vi "Compute Convolution 32f.vi"(8 "Error In":errorcluster, 10 "Input Memory":T4 {"Dimension"."Width" min=1; "Dimension"."Height" min=1; "Dimension"."Depth" min=1}, 11 "Convolution Object":T1 {"Convolved Memory Object"."Dimension"."Width" min=1; "Convolved Memory Object"."Dimension"."Height" min=1; "Convolved Memory Object"."Dimension"."Depth" min=1; "Kernel Memory Object"."Dimension"."Width" min=1; "Kernel Memory Object"."Dimension"."Height" min=1; "Kernel Memory Object"."Dimension"."Depth" min=1}) -> (0 "Error Out":errorcluster, 2 "Convolved Memory":T4 {"Dimension"."Width" min=1; "Dimension"."Height" min=1; "Dimension"."Depth" min=1}, 3 "Convolution Object Out":T1 {"Convolved Memory Object"."Dimension"."Width" min=1; "Convolved Memory Object"."Dimension"."Height" min=1; "Convolved Memory Object"."Dimension"."Depth" min=1; "Kernel Memory Object"."Dimension"."Width" min=1; "Kernel Memory Object"."Dimension"."Height" min=1; "Kernel Memory Object"."Dimension"."Depth" min=1}, 4 "Time in ms":dbl)   [LabVIEW 2012, in "OpenCLV x64.lvlib"]
doc: "Convolves the input memory object with the kernel that has been previously set. The output is seperate from the input."
uses:
  OpenCLV x64.lvlib
  Controls/Convolution Object.ctl
  Controls/Device ID.ctl
  Controls/Program Handle.ctl
  Controls/Memory Object.ctl
  Controls/Memory ID.ctl
  User Controls/Array Dimensions.ctl
  Controls/Memory Type.ctl
  Error Checking/Add Error Functional Global.vi
  Set Kernel Arguments/Set Kernel Arguments Memory Object.vi
  Set Kernel Arguments/Set Kernel Arguments int.vi
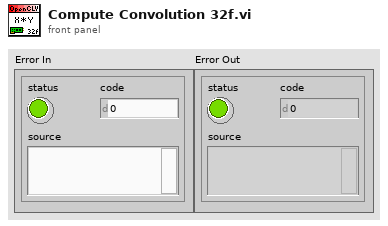
[diagram p1: front panel]
types:
  T1 = typedef "OpenCLV x64.lvlib/Convolution Object.ctl" = cluster{"Device In":T2, "Program Handle":T3, "Kernel Memory Object":T4, "Convolved Memory Object":T4}
  T2 = typedef "OpenCLV x64.lvlib/Device ID.ctl" = u64
  T3 = typedef "OpenCLV x64.lvlib/Program Handle.ctl" = u64
  T4 = typedef "OpenCLV x64.lvlib/Memory Object.ctl" = cluster{"Device ID":T2, "Memeroy ID":T5, "Dimension":T6, "Memory Type":T7}
  T5 = typedef "OpenCLV x64.lvlib/Memory ID.ctl" = u64
  T6 = typedef "Array Dimensions.ctl" = cluster{"Depth":u64, "Height":u64, "Width":u64}
  T7 = typedef "OpenCLV x64.lvlib/Memory Type.ctl" = enum16{"32f", "u8", "i8", "u16", "i16", "u32", "i32", "64f"}
  T8 = typedef "OpenCLV x64.lvlib/Kernel Handle.ctl" = u64
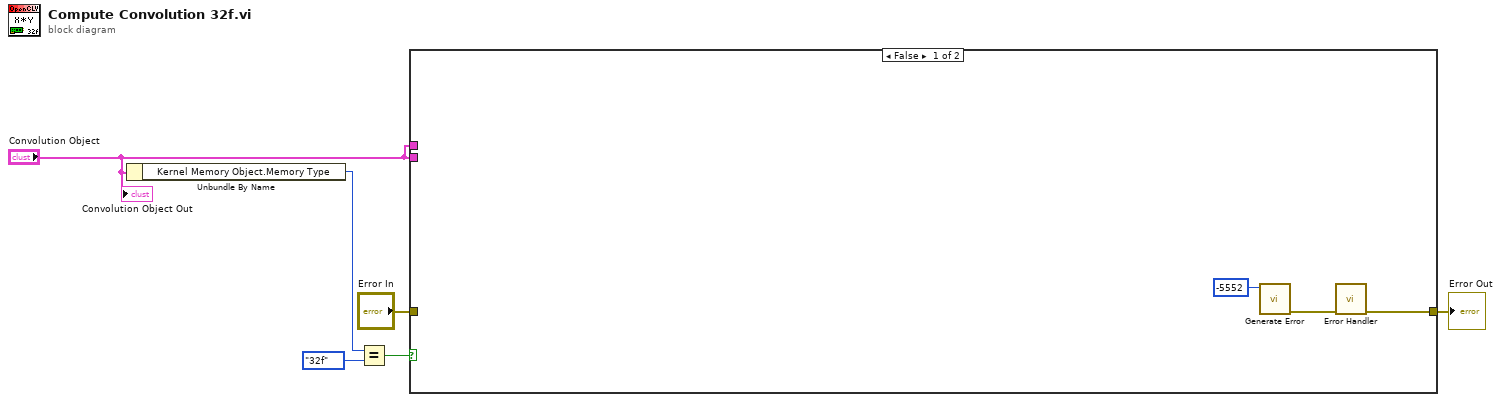
[diagram p0: block diagram]
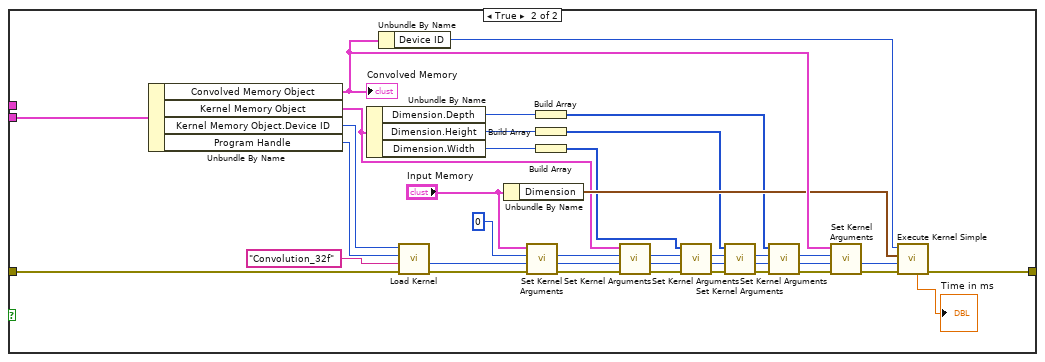
[diagram p2: hidden frame]
diagram:
  n1 = Unbundle By Name("Convolution Object") -> ("Kernel Memory Object.Memory Type"=w6:T7)
  n2 = Equal?(x=w6, y=Memory_Type."32f") -> (x = y?=w5:bool)
  n3 = case shown="False" w5 {
    tunnel: [w7 w46] -> w2
    tunnel: "Convolution Object" -> [_ w36]
    tunnel: "Error In" -> [_ w47]
    tunnel: "Convolution Object" -> [_ _]
    frame False {
      n4 = call "Generate Error.vi"("Error"=-5552) -> ("error out"=w8:errorcluster)  [unwired: 10 in]
      n5 = call-poly "Error Handler.vi"("Error In"=w8) -> ("Error Out"=w7:errorcluster)  [unwired: 10 in]
    }
    frame True {
      n6 = Unbundle By Name(w36) -> ("Convolved Memory Object"=w31:T4, "Kernel Memory Object"=w28:T4, "Kernel Memory Object.Device ID"=w45:T2, "Program Handle"=w35:T3)
      "Convolved Memory" <- w31
      n7 = Unbundle By Name(w28) -> ("Dimension.Depth"=w14:u64, "Dimension.Height"=w19:u64, "Dimension.Width"=w23:u64)
      n8 = Unbundle By Name(w31) -> ("Device ID"=w30:T2)
      n9 = call "Load Kernel.vi"("Error In"=w47, "Kernel Name"="Convolution_32f", "Program Handle"=w35, "Device In"=w45) -> ("Error Out"=w43:errorcluster, "Kernel Handle"=w42:T8)  [unwired: 4 in, 2 out]
      n10 = Unbundle By Name("Input Memory") -> ("Dimension"=w29:T6)
      n11 = call-poly "Set Kernel Arguments.vi"("Error In"=w43, "Kernel Handle"=w42, "Argument Number"=0, "Memory Object"="Input Memory") -> ("Error Out"=w40:errorcluster, "Kernel Handle out"=w39:T8, "Auto Inc Arugment Number"=w38:i32)  [unwired: 5 in]
      n12 = Build Array(w14) -> (w13:u64[])
      n13 = Build Array(w19) -> (w18:u64[])
      n14 = Build Array(w23) -> (w24:u64[])
      n15 = call-poly "Set Kernel Arguments.vi"("Error In"=w40, "Kernel Handle"=w39, "Argument Number"=w38, "Memory Object"=w28) -> ("Error Out"=w27:errorcluster, "Kernel Handle out"=w26:T8, "Auto Inc Arugment Number"=w25:i32)  [unwired: 5 in]
      n16 = call-poly "Set Kernel Arguments.vi"("Error In"=w27, "Kernel Handle"=w26, "Argument Number"=w25, "i32 Constant"=w24) -> ("Error Out"=w22:errorcluster, "Kernel Handle out"=w21:T8, "Auto Inc Arugment Number"=w20:i32)  [unwired: 5 in]
      n17 = call-poly "Set Kernel Arguments.vi"("Error In"=w22, "Kernel Handle"=w21, "Argument Number"=w20, "i32 Constant"=w18) -> ("Error Out"=w17:errorcluster, "Kernel Handle out"=w16:T8, "Auto Inc Arugment Number"=w15:i32)  [unwired: 5 in]
      n18 = call-poly "Set Kernel Arguments.vi"("Error In"=w17, "Kernel Handle"=w16, "Argument Number"=w15, "i32 Constant"=w13) -> ("Error Out"=w12:errorcluster, "Kernel Handle out"=w11:T8, "Auto Inc Arugment Number"=w10:i32)  [unwired: 5 in]
      n19 = call-poly "Set Kernel Arguments.vi"("Error In"=w12, "Kernel Handle"=w11, "Argument Number"=w10, "Memory Object"=w31) -> ("Error Out"=w34:errorcluster, "Kernel Handle out"=w33:T8)  [unwired: 5 in, 1 out]
      n20 = call "Execute Kernel Simple.vi"("Error In"=w34, "Kernel Handle"=w33, "Thread Dimensions"=w29, "Device In"=w30) -> ("Error Out"=w46:errorcluster, "Time in ms"=→"Time in ms":dbl)  [unwired: 4 in, 2 out]
    }
  }
  "Error Out" <- w2
  "Convolution Object Out" <- "Convolution Object"
